vi "Eq. Tiempo.vi"(1 "Día del año (n)":dbl) -> (0 "Eq. Tiempo":dbl)   [LabVIEW 2020]
panel:
  out "Segundos":i32
  out "Minutos":i32
  out "Grados":i32
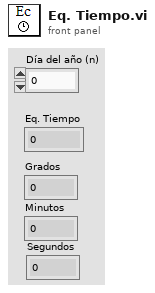
[diagram p1: front panel]
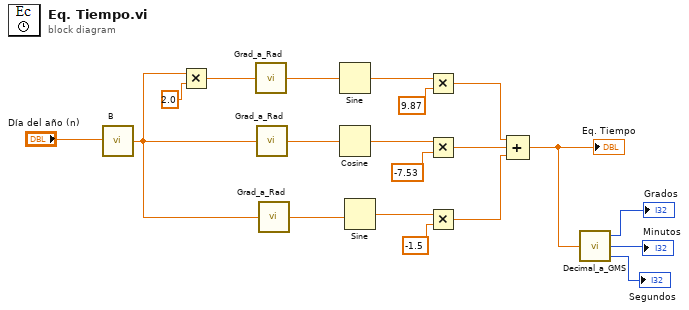
[diagram p0: block diagram]
diagram:
  n1 = call "B.vi"("n"="Día del año (n)") -> ("B"=w14:dbl)
  n2 = Multiply(x=w14, y=2.0) -> (x*y=w15:dbl)
  n3 = call "Grad_a_Rad.vi"("Grados"=w15) -> ("Radianes"=w20:dbl)
  n4 = call "Grad_a_Rad.vi"("Grados"=w14) -> ("Radianes"=w19:dbl)
  n5 = call "Grad_a_Rad.vi"("Grados"=w14) -> ("Radianes"=w18:dbl)
  n6 = Sine(x=w20) -> (sin(x)=w8:dbl)
  n7 = Cosine(x=w19) -> (cos(x)=w10:dbl)
  n8 = Sine(x=w18) -> (sin(x)=w12:dbl)
  n9 = Multiply(x=w8, y=9.87) -> (x*y=w7:dbl)
  n10 = Multiply(x=w10, y=-7.53) -> (x*y=w6:dbl)
  n11 = Multiply(x=w12, y=-1.5) -> (x*y=w5:dbl)
  n12 = Compound Arithmetic op=ADD(w7, w6, w5) -> (w4:dbl)
  "Eq. Tiempo" <- w4
  n13 = call "Decimal_a_GMS.vi"("Decimal"=w4) -> ("Grados"=→"Grados":i32, "Minutos"=→"Minutos":i32, "Segundos"=→"Segundos":i32)
